vi "REFERECECONNECTEUR.vi"(9 "nombre de piéce":string, 11 "compteur":i32) -> (0 "error out":errorcluster)   [LabVIEW 2021]
uses:
  <vilib>/Utility/file.llb/Write Delimited Spreadsheet (string).vi
  <vilib>/Utility/file.llb/Write Delimited Spreadsheet (I64).vi
panel:
  out "new file path (Not A Path if cancelled)":path
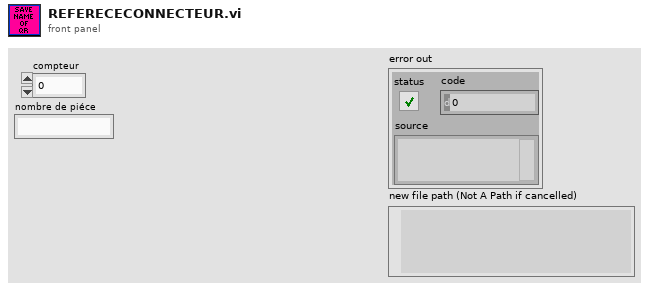
[diagram p1: front panel]
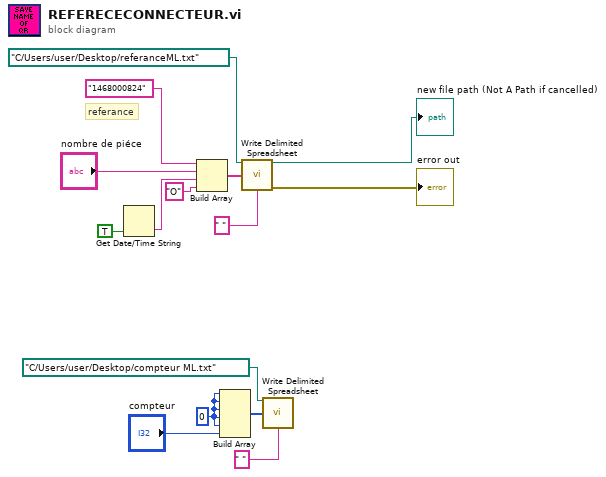
[diagram p0: block diagram]
diagram:
  w8 = 0
  # "referance"
  n1 = Get Date/Time String(want seconds? (F)=TRUE) -> (time string=w6:string)  [unwired: 2 in, 1 out]
  n2 = Build Array("1468000824" ("element"), "nombre de piéce", w6, "O" ("element")) -> (w10:string[])
  n3 = Build Array(w8, w8, w8, w8, w8, "compteur") -> (w9:i32[])
  n4 = call-poly <vilib>:"Write Delimited Spreadsheet.vi"("file path (dialog if empty)"=path "C:/Users/user/Desktop/referanceML.txt", "1D data"=w10, "delimiter (\\t)"=" " ("delimiter (\\t)")) -> ("new file path (Not A Path if cancelled)"=→"new file path (Not A Path if cancelled)":path, "error out"=→"error out":errorcluster)  [unwired: 11 in]
  n5 = call-poly <vilib>:"Write Delimited Spreadsheet.vi"("file path (dialog if empty)"=path "C:/Users/user/Desktop/compteur ML.txt", "1D data"=w9, "delimiter (\\t)"=" " ("delimiter (\\t)")) -> ()  [unwired: 11 in, 2 out]
